vi "ControlStop.vi"(3 "error in (no error)":errorcluster, 5 "Task ID":u32) -> (0 "error out":errorcluster, 2 "Task ID":u32)   [LabVIEW 2015]
uses:
  Windows/System32/AdvLvDaq.dll
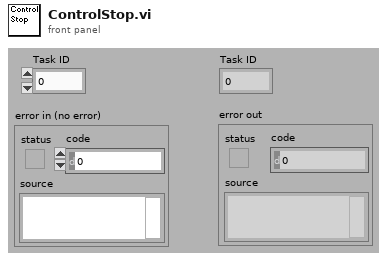
[diagram p1: front panel]
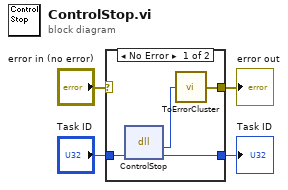
[diagram p0: block diagram]
diagram:
  n1 = case shown="No Error" "error in (no error)" {
    selector: "error in (no error)" -> [_ w9]
    tunnel: "Task ID" -> [w8 w10]
    tunnel: [w7 w10] -> w2
    tunnel: [w5 w9] -> w1
    frame No Error {
      n2 = dll-call lib="C:/Windows/System32/AdvLvDaq.dll" fn="ControlStop"("taskId"=w8) -> ("return type"=w6:i32, "taskId"=w7:u32)  [unwired: 3 in, 2 out]
      n3 = call "ToErrorCluster.vi"("error code"=w6) -> ("error out"=w5:errorcluster)
    }
    frame Error {
    }
  }
  "error out" <- w1
  "Task ID" <- w2
